vi "Automation(Feedback without use switch).vi"() -> ()   [LabVIEW 2015]
panel:
  out "Automation(Feedback without use switch)":bool
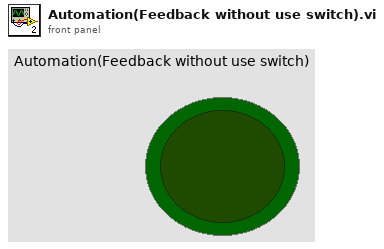
[diagram p1: front panel]
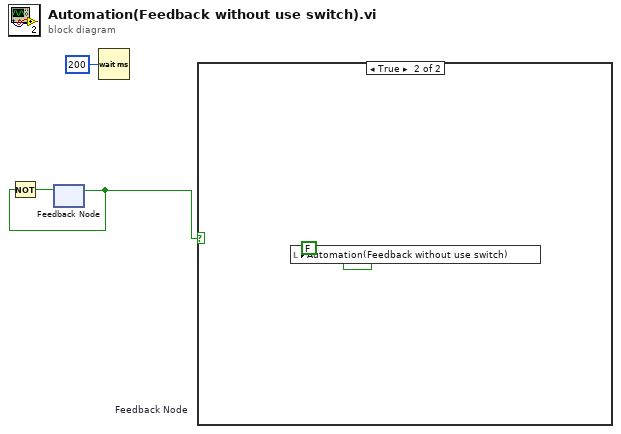
[diagram p0: block diagram]
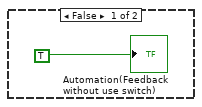
[diagram p2: hidden frame]
diagram:
  n1 = feedback #1 "Feedback Node"() -> (w2:bool)  [unwired: 1 in]
  n2 = Not(x=w2) -> (.not. x?=w3:bool)
  n3 = feedback-in #1(w3) -> ()
  n4 = Wait (ms)(milliseconds to wait=u32 200) -> ()  [unwired: 1 out]
  n5 = case shown="True" w2 {
    frame False {
      "Automation(Feedback without use switch)" <- TRUE
    }
    frame True {
      n6 = local write "Automation(Feedback without use switch)"(FALSE) -> ()
    }
  }
